vi "drivetrain.vi"(2 "Sensors":cluster{"Left Encoder":dbl, "Right Encoder":dbl}, 3 "CurrentStatusArray":bool[][](array[boolean]), 4 "Checkmarks Array":bool[][](array[boolean])) -> (0 "CurrentStatusArray Output":bool[][](array[boolean]), 1 "Checkmarks Array Output":bool[][](array[boolean]))   [LabVIEW 2011]
panel:
  in  "EncoderVelocityDeadband":dbl
  in  "HighGearEncoder Constant":dbl
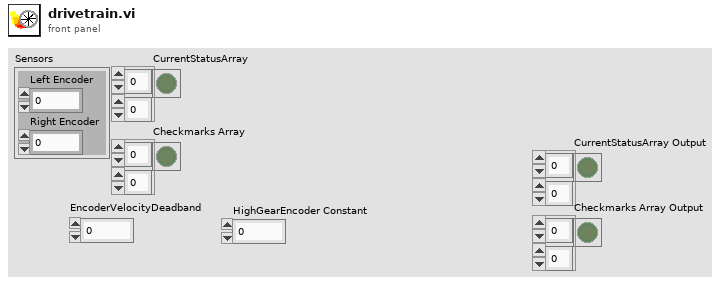
[diagram p1: front panel]
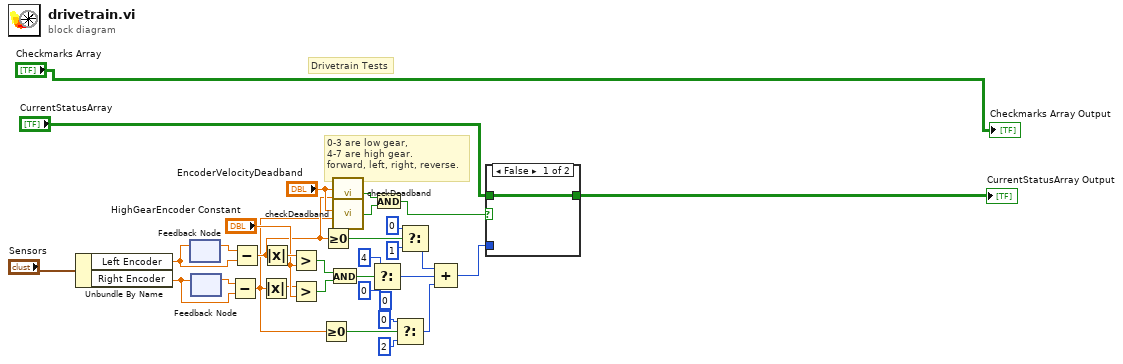
[diagram p0: block diagram]
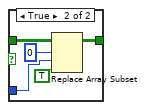
[diagram p2: hidden frame]
diagram:
  (unwired) i8 0 ("t")
  # "Drivetrain Tests"
  # "0-3 are low gear,\n4-7 are high gear.\nforward, left, right, reverse."
  n1 = Unbundle By Name("Sensors") -> ("Left Encoder"=w31:dbl, "Right Encoder"=w3:dbl)
  n2 = feedback #1() -> (w32:dbl)  [unwired: 1 in]
  n3 = feedback-in #1(w31) -> ()
  n4 = feedback #2() -> (w30:dbl)  [unwired: 1 in]
  n5 = feedback-in #2(w3) -> ()
  n6 = Subtract(x=w30, y=w3) -> (x-y=w6:dbl)
  n7 = Subtract(x=w32, y=w31) -> (x-y=w11:dbl)
  n8 = Absolute Value(x=w6) -> (abs(x)=w27:dbl)
  n9 = Absolute Value(x=w11) -> (abs(x)=w29:dbl)
  n10 = Greater?(x=w29, y="HighGearEncoder Constant") -> (0:w23:bool)
  n11 = Greater?(x=w27, y="HighGearEncoder Constant") -> (0:w22:bool)
  n12 = Greater Or Equal To 0?(x=w6) -> (x >= 0?=w7:bool)
  n13 = Greater Or Equal To 0?(x=w11) -> (x >= 0?=w20:bool)
  n14 = And(x=w23, y=w22) -> (x .and. y?=w26:bool)
  n15 = call "checkDeadband.vi"("tolerance"="EncoderVelocityDeadband", "input"=w11) -> ("output"=w14:bool)  [unwired: 5 in]
  n16 = call "checkDeadband.vi"("tolerance"="EncoderVelocityDeadband", "input"=w6) -> ("output"=w13:bool)  [unwired: 5 in]
  n17 = Select(t=i8 4, s=w26, f=i8 0) -> (s? t:f=w21:i8)
  n18 = And(x=w14, y=w13) -> (x .and. y?=w10:bool)
  n19 = Select(t=i8 0, s=w7, f=i8 2) -> (s? t:f=w17:i8)
  n20 = Select(t=i8 0, s=w20, f=i8 1) -> (s? t:f=w16:i8)
  n21 = Compound Arithmetic op=ADD(w16, w21, w17) -> (w15:i8)
  n22 = case shown="False" w10 {
    tunnel: "CurrentStatusArray" -> [w33 w38]
    tunnel: w15 -> [_ w34]
    tunnel: [w33 w35] -> w2
    frame False {
    }
    frame True {
      n23 = Replace Array Subset(array=w38, new element=TRUE ("new element/subarray"), index (row)=0, index (col)=w34) -> (w35:bool[][])
    }
  }
  "CurrentStatusArray Output" <- w2
  "Checkmarks Array Output" <- "Checkmarks Array"
